vi "PWM.vi"(0 "Count(Ticks)":u32 caption="Hz", 8 "Pluse":u32) -> ()   [LabVIEW 2018]
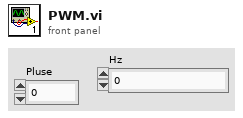
[diagram p1: front panel]
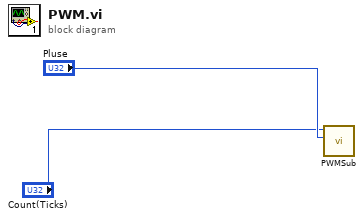
[diagram p0: block diagram]
diagram:
  n1 = call "PWMSub.vi"("Pluse"="Pluse", "Count(Ticks)"="Count(Ticks)") -> ()  [unwired: 10 in]
